vi "log analysis_gps.vi"() -> ()   [LabVIEW 2018] (continued)
INS_ALIGNMENT_COMPLETE,INS_RTKFIXED,37.37088132753,126.72154143045,8.4401,22.3000,-0.3278,-0.2536,0.0246,-0.732605001,0.589727641,213.014456450,0.4341,0.3007,0.5858,0.1132,0.0942,0.0801,0.0958,0.0999,5.1140,0f000001,0*274257ec\n\tsystem status\tnormal 2 27.800000 0 0\trobot status\t62.565143\t83.363741\t8.440100\t-0.732605\t0.589728\t-123.014456\t0.484000\t-0.004000\n\t\n15:50:00.3\tlog_raw\tgps_raw\t#INSPVAXA,USB3,0,42.0,FINESTEERING,2107,283818.350,02000000,471d,15824;INS_ALIGNMENT_COMPLETE,INS_RTKFIXED,37.37087991199,126.72154012021,8.4416,22.3000,-0.1368,-0.1470,0.0384,-0.668714112,0.493381563,212.999632348,0.4348,0.3009,0.5860,0.1136,0.0943,0.0809,0.0957,0.0999,5.1129,0f000001,0*1003161e\n\tsystem status\tnormal 2 27.800000 0 0\trobot status\t62.449084\t83.206639\t8.441600\t-0.668714\t0.493382\t-122.999632\t0.347000\t0.082000\n\t\n15:50:00.8\tlog_raw\tgps_raw\t#INSPVAXA,USB3,0,42.0,FINESTEERING,2107,283818.850,02000000,471d,15824;INS_ALIGNMENT_COMPLETE,INS_RTKFIXED,37.37087810564,126.72153855101,8.4445,22.3000,-0.4167,-0.3108,0.0271,-0.967030857,0.764287443,212.987620648,0.4348,0.3009,0.5860,0.1136,0.0943,0.0809,0.0957,0.0999,5.1129,0f000001,0*cade7f0f\n\tsystem status\tnormal 2 27.800000 0 0\trobot status\t62.310087\t83.006163\t8.444500\t-0.967031\t0.764287\t-122.987621\t0.541000\t-0.038000\n\t\n15:50:01.3\tlog_raw\tgps_raw\t\tsystem status\tnormal 2 27.700000 0 0\trobot status\t62.183899\t82.831063\t8.448200\t-1.040887\t0.633536\t-122.852792\t0.541000\t-0.102000\n\t\n15:50:01.8\tlog_raw\tgps_raw\t#INSPVAXA,USB3,0,48.0,FINESTEERING,2107,283819.850,02008000,471d,15824;INS_ALIGNMENT_COMPLETE,INS_RTKFIXED,37.37087469725,126.72153545428,8.4519,22.3000,-0.3206,-0.2482,0.0337,-0.732742938,0.483764401,213.124733025,0.4356,0.3015,0.5865,0.1140,0.0945,0.0816,0.0957,0.0999,5.1129,0f000001,0*fd809d66\n\tsystem status\tnormal 2 27.800000 0 0\trobot status\t62.035784\t82.627886\t8.451900\t-0.732743\t0.483764\t-123.124733\t0.474000\t-0.007000\n\t\n15:50:02.3\tlog_raw\tgps_raw\t#INSPVAXA,USB3,0,50.0,FINESTEERING,2107,283820.350,02008000,471d,15824;INS_ALIGNMENT_COMPLETE,INS_RTKFIXED,37.37087296887,126.72153391310,8.4559,22.3000,-0.3682,-0.2755,0.0355,-0.960553377,0.385725607,213.158574943,0.4360,0.3020,0.5871,0.1135,0.0940,0.0814,0.0957,0.0998,5.1132,0f000001,0*75b28094\n\tsystem status\tnormal 2 27.800000 0 0\trobot status\t61.899269\t82.436064\t8.455900\t-0.960553\t0.385726\t-123.158575\t0.505000\t0.011000\n\t\n15:50:02.8\tlog_raw\tgps_raw\t#INSPVAXA,USB3,0,50.0,FINESTEERING,2107,283820.850,02008000,471d,15824;INS_ALIGNMENT_COMPLETE,INS_RTKFIXED,37.37087124768,126.72153233501,8.4599,22.3000,-0.3422,-0.2623,0.0223,-0.701545718,0.294421215,213.284375134,0.4360,0.3020,0.5871,0.1135,0.0940,0.0814,0.0957,0.0998,5.1132,0f000001,0*60222fab\n\tsystem status\tnormal 2 27.800000 0 0\trobot status\t61.759484\t82.245039\t8.459900\t-0.701546\t0.294421\t-123.284375\t0.485000\t-0.013000\n\t\n15:50:03.3\tlog_raw\tgps_raw\t\tsystem status\tnormal 2 27.800000 0 0\trobot status\t61.620063\t82.053533\t8.464300\t-0.588483\t0.601593\t-123.330057\t0.501000\t-0.003000\n\t\n15:50:03.8\tlog_raw\tgps_raw\t\tsystem status\tnormal 2 27.800000 0 0\trobot status\t61.480841\t81.860839\t8.467500\t-0.490654\t0.559524\t-123.370986\t0.492000\t0.000000\n\t\n15:50:04.3\tlog_raw\tgps_raw\t#INSPVAXA,USB3,0,47.5,FINESTEERING,2107,283822.350,02008000,471d,15824;INS_ALIGNMENT_COMPLETE,INS_RTKFIXED,37.37086605631,126.72152760376,8.4704,22.3000,-0.3621,-0.2743,0.0261,-0.283958225,0.746560845,213.501890375,0.4357,0.3020,0.5877,0.1128,0.0932,0.0807,0.0958,0.0999,5.1149,0f000001,0*0669f83a\n\tsystem status\tnormal 2 27.800000 0 0\trobot status\t61.340398\t81.668880\t8.470400\t-0.283958\t0.746561\t-123.501890\t0.502000\t0.003000\n\t\n15:50:04.8\tlog_raw\tgps_raw\t#INSPVAXA,USB3,0,47.5,FINESTEERING,2107,283822.850,02008000,471d,15824;INS_ALIGNMENT_COMPLETE,INS_RTKFIXED,37.37086430536,126.72152600341,8.4729,22.3000,-0.3685,-0.2624,0.0208,-0.369026169,0.243772602,213.702415244,0.4357,0.3020,0.5877,0.1128,0.0932,0.0807,0.0958,0.0999,5.1149,0f000001,0*05a2b3f5\n\tsystem status\tnormal 2 27.800000 0 0\trobot status\t61.198641\t81.474552\t8.472900\t-0.369026\t0.243773\t-123.702415\t0.487000\t-0.013000\n\t\n15:50:05.3\tlog_raw\tgps_raw\t#INSPVAXA,USB3,0,51.5,FINESTEERING,2107,283823.350,02000000,471d,15824;INS_ALIGNMENT_COMPLETE,INS_RTKFIXED,37.37086260441,126.72152443604,8.4782,22.3000,-0.3582,-0.2656,0.0432,-0.497136063,0.605287722,213.732183523,0.4353,0.3025,0.5877,0.1126,0.0930,0.0805,0.0959,0.0999,5.1164,0f000001,0*99f3cfc8\n\tsystem status\tnormal 2 27.800000 0 0\trobot status\t61.059806\t81.285774\t8.478200\t-0.497136\t0.605288\t-123.732184\t0.485000\t-0.006000\n\t\n15:50:05.8\tlog_raw\tgps_raw\t\tsystem status\tnormal 2 27.800000 0 0\trobot status\t60.916983\t81.093453\t8.482200\t-0.454568\t0.858400\t-123.956914\t0.505000\t-0.014000\n\t\n15:50:06.3\tlog_raw\tgps_raw\t\tsystem status\tnormal 2 27.800000 0 0\trobot status\t60.774020\t80.901518\t8.486300\t-0.505119\t0.869567\t-124.073928\t0.475000\t-0.001000\n\t\n15:50:06.8\tlog_raw\tgps_raw\t\tsystem status\tnormal 2 27.800000 0 0\trobot status\t60.629827\t80.709035\t8.491500\t-0.511995\t0.882241\t-124.119289\t0.499000\t0.008000\n\t\n15:50:07.3\tlog_raw\tgps_raw\t\tsystem status\tnormal 2 27.800000 0 0\trobot status\t60.486737\t80.520026\t8.496700\t-0.379564\t1.020699\t-124.239157\t0.501000\t0.000000\n\t\n15:50:07.8\tlog_raw\tgps_raw\t\tsystem status\tnormal 2 27.800000 0 0\trobot status\t60.338417\t80.322446\t8.499300\t-0.432771\t0.777061\t-124.291372\t0.483000\t0.003000\n\t\n15:50:08.3\tlog_raw\tgps_raw\t#INSPVAXA,USB3,0,50.0,FINESTEERING,2107,283826.350,02000000,471d,15824;INS_ALIGNMENT_COMPLETE,INS_RTKFIXED,37.37085224696,126.72151466397,8.5036,22.3000,-0.3609,-0.2791,0.0409,-0.133797163,0.866362629,214.216095146,0.4345,0.3034,0.5878,0.1129,0.0936,0.0804,0.0960,0.1000,5.1194,0f000001,0*7d577a89\n\tsystem status\tnormal 2 27.700000 0 0\trobot status\t60.194212\t80.136263\t8.503600\t-0.133797\t0.866363\t-124.216095\t0.510000\t0.000000\n\t\n15:50:08.8\tlog_raw\tgps_raw\t#INSPVAXA,USB3,0,50.0,FINESTEERING,2107,283826.850,02000000,471d,15824;INS_ALIGNMENT_COMPLETE,INS_RTKFIXED,37.37085047497,126.72151297785,8.5076,22.3000,-0.3736,-0.2676,0.0140,-0.059092232,0.621746076,214.361721087,0.4345,0.3034,0.5878,0.1129,0.0936,0.0804,0.0960,0.1000,5.1194,0f000001,0*1a2aa4a2\n\tsystem status\tnormal 2 27.800000 0 0\trobot status\t60.044859\t79.939600\t8.507600\t-0.059092\t0.621746\t-124.361721\t0.500000\t0.002000\n\t\n15:50:09.3\tlog_raw\tgps_raw\t\tsystem status\tnormal 2 27.800000 0 0\trobot status\t59.900989\t79.749781\t8.510000\t-0.117922\t0.897612\t-124.301125\t0.496000\t0.007000\n\t\n15:50:09.8\tlog_raw\tgps_raw\t\tsystem status\tnormal 2 27.800000 0 0\trobot status\t59.753594\t79.555314\t8.514600\t-0.246147\t0.942410\t-124.362581\t0.504000\t0.012000\n\t\n15:50:10.3\tlog_raw\tgps_raw\t\tsystem status\tnormal 2 27.700000 0 0\trobot status\t59.607367\t79.367106\t8.518000\t-0.100537\t0.892414\t-124.256179\t0.571000\t-0.106000\n\t\n15:50:10.8\tlog_raw\tgps_raw\t#INSPVAXA,USB3,0,47.0,FINESTEERING,2107,283828.850,02000000,471d,15824;INS_ALIGNMENT_COMPLETE,INS_RTKFIXED,37.37084355919,126.72150637181,8.5210,22.3000,-0.3615,-0.2654,0.0256,-0.407156053,0.613221489,214.165441320,0.4336,0.3030,0.5876,0.1126,0.0934,0.0800,0.0960,0.1000,5.1212,0f000001,0*2be625c6\n\tsystem status\tnormal 2 27.700000 0 0\trobot status\t59.459706\t79.172059\t8.521000\t-0.407156\t0.613221\t-124.165441\t0.420000\t0.099000\n\t\n15:50:11.3\tlog_raw\tgps_raw\t\tsystem status\tnormal 2 27.800000 0 0\trobot status\t59.313902\t78.981500\t8.523300\t-0.458738\t0.721026\t-124.084724\t0.444000\t0.089000\n\t\n15:50:11.8\tlog_raw\tgps_raw\t\tsystem status\tnormal 2 27.700000 0 0\trobot status\t59.170415\t78.788865\t8.523100\t-0.646434\t0.705143\t-123.927806\t0.431000\t0.105000\n\t\n15:50:12.3\tlog_raw\tgps_raw\t\tsystem status\tnormal 2 27.800000 0 0\trobot status\t59.029369\t78.598762\t8.525600\t-0.727661\t0.618524\t-123.799711\t0.573000\t-0.111000\n\t\n15:50:12.8\tlog_raw\tgps_raw\t\tsystem status\tnormal 2 27.800000 0 0\trobot status\t58.884800\t78.404387\t8.527700\t-0.829758\t0.768744\t-123.767439\t0.440000\t0.084000\n\t\n15:50:13.3\tlog_raw\tgps_raw\t\tsystem status\tnormal 2 27.800000 0 0\trobot status\t58.743546\t78.215101\t8.526800\t-0.859789\t0.544559\t-123.753093\t0.569000\t-0.115000\n\t\n15:50:13.8\tlog_raw\tgps_raw\t\tsystem status\tnormal 2 27.800000 0 0\trobot status\t58.600898\t78.024369\t8.526600\t-0.696753\t0.469479\t-123.492403\t0.470000\t0.049000\n\t\n15:50:14.3\tlog_raw\tgps_raw\t\tsystem status\tnormal 2 27.700000 0 0\trobot status\t58.467877\t77.847457\t8.526300\t-0.753284\t0.477673\t-123.294500\t0.540000\t-0.104000\n\t\n15:50:14.8\tlog_raw\tgps_raw\t\tsystem status\tnormal 2 27.800000 0 0\trobot status\t58.320241\t77.650801\t8.527400\t-0.419843\t0.351195\t-123.324600\t0.447000\t0.018000\n\t\n15:50:15.3\tlog_raw\tgps_raw\t#INSPVAXA,USB3,0,49.5,FINESTEERING,2107,283833.350,02000000,471d,15824;INS_ALIGNMENT_COMPLETE,INS_RTKFIXED,37.37082814557,126.72149191799,8.5253,22.3000,-0.3988,-0.2653,0.0143,-0.599400887,0.523128391,213.276992929,0.4351,0.3016,0.5901,0.1136,0.0943,0.0827,0.0961,0.1001,5.1237,0f000001,0*dafc27db\n\tsystem status\tnormal 2 27.800000 0 0\trobot status\t58.179411\t77.461394\t8.525300\t-0.599401\t0.523128\t-123.276993\t0.615000\t-0.169000\n\t\n15:50:15.8\tlog_raw\tgps_raw\t\tsystem status\tnormal 2 27.700000 0 0\trobot status\t58.040086\t77.274601\t8.523600\t-0.642218\t0.408269\t-123.044870\t0.478000\t0.045000\n\t\n15:50:16.3\tlog_raw\tgps_raw\t\tsystem status\tnormal 2 27.700000 0 0\trobot status\t57.897701\t77.084219\t8.524200\t-0.645532\t0.325284\t-123.014654\t0.427000\t0.080000\n\t\n15:50:16.9\tlog_raw\tgps_raw\t\tsystem status\tnormal 2 27.800000 0 0\trobot status\t57.755522\t76.892077\t8.525700\t-0.812673\t0.258621\t-122.912534\t0.599000\t-0.151000\n\t\n15:50:17.4\tlog_raw\tgps_raw\t\tsystem status\tnormal 2 27.800000 0 0\trobot status\t57.615508\t76.704244\t8.527300\t-0.871477\t0.465364\t-122.750872\t0.437000\t0.097000\n\t\n15:50:17.8\tlog_raw\tgps_raw\t\tsystem status\tnormal 2 27.800000 0 0\trobot status\t57.474420\t76.516325\t8.527900\t-0.830453\t0.488115\t-122.693748\t0.441000\t0.077000\n\t\n15:50:18.3\tlog_raw\tgps_raw\t\tsystem status\tnormal 2 27.700000 0 0\trobot status\t57.335246\t76.328739\t8.530900\t-1.116689\t0.751675\t-122.684563\t0.468000\t0.035000\n\t\n15:50:18.9\tlog_raw\tgps_raw\t\tsystem status\tnormal 2 27.700000 0 0\trobot status\t57.194986\t76.142393\t8.532800\t-1.080685\t0.717974\t-122.524301\t0.445000\t0.006000\n\t\n15:50:19.4\tlog_raw\tgps_raw\t\tsystem status\tnormal 2 27.700000 0 0\trobot status\t57.069798\t75.976583\t8.534400\t-1.000976\t0.803716\t-122.391423\t0.541000\t0.029000\n\t\n15:50:19.9\tlog_raw\tgps_raw\t\tsystem status\tnormal 2 27.800000 0 0\trobot status\t56.929080\t75.785380\t8.534800\t-1.060163\t0.551148\t-122.452254\t0.510000\t-0.067000\n\t\n15:50:20.4\tlog_raw\tgps_raw\t\tsystem status\tnormal 2 27.800000 0 0\trobot status\t56.786562\t75.588482\t8.537500\t-1.255740\t0.371969\t-122.455535\t0.455000\t0.052000\n\t\n15:50:20.9\tlog_raw\tgps_raw\t\tsystem status\tnormal 2 27.800000 0 0\trobot status\t56.646511\t75.399961\t8.540500\t-0.936257\t0.326700\t-122.440428\t0.521000\t-0.009000\n\t\n15:50:21.4\tlog_raw\tgps_raw\t\tsystem status\tnormal 2 27.800000 0 0\trobot status\t56.509252\t75.212453\t8.543000\t-0.983282\t0.423992\t-122.415900\t0.506000\t0.009000\n\t\n15:50:21.9\tlog_raw\tgps_raw\t\tsystem status\tnormal 2 27.800000 0 0\trobot status\t56.370098\t75.020504\t8.546300\t-1.075445\t0.704997\t-122.497458\t0.489000\t0.003000\n\t\n15:50:22.4\tlog_raw\tgps_raw\t\tsystem status\tnormal 2 27.800000 0 0\trobot status\t56.230758\t74.831082\t8.551300\t-0.784818\t1.051226\t-122.242457\t0.562000\t-0.121000\n\t\n15:50:22.9\tlog_raw\tgps_raw\t\tsystem status\tnormal 2 27.700000 0 0\trobot status\t56.089782\t74.634051\t8.555400\t-0.965192\t0.771989\t-122.204085\t0.418000\t0.096000\n\t\n15:50:23.4\tlog_raw\tgps_raw\t\tsystem status\tnormal 2 27.700000 0 0\trobot status\t55.952267\t74.442660\t8.561500\t-1.095253\t0.958840\t-121.984787\t0.476000\t0.048000\n\t\n15:50:23.9\tlog_raw\tgps_raw\t\tsystem status\tnormal 2 27.800000 0 0\trobot status\t55.810060\t74.249698\t8.568200\t-0.625932\t0.756695\t-121.962841\t0.491000\t0.012000\n\t\n15:50:24.4\tlog_raw\tgps_raw\t\tsystem status\tnormal 2 27.700000 0 0\trobot status\t55.672258\t74.056371\t8.572700\t-0.978139\t0.659965\t-121.899886\t0.414000\t0.093000\n\t\n15:50:24.9\tlog_raw\tgps_raw\t\tsystem status\tnormal 2 27.800000 0 0\trobot status\t55.531120\t73.861309\t8.578200\t-0.929865\t0.602313\t-121.836312\t0.576000\t-0.107000\n\t\n15:50:25.4\tlog_raw\tgps_raw\t\tsystem status\tnormal 2 27.800000 0 0\trobot status\t55.387324\t73.664243\t8.582300\t-0.402762\t0.316758\t-121.817690\t0.484000\t0.008000\n\t\n15:50:25.9\tlog_raw\tgps_raw\t\tsystem status\tnormal 2 27.800000 0 0\trobot status\t55.250271\t73.472188\t8.586400\t-0.565675\t0.466930\t-121.851880\t0.493000\t0.003000\n\t\n15:50:26.4\tlog_raw\tgps_raw\t\tsystem status\tnormal 2 27.800000 0 0\trobot status\t55.106611\t73.274986\t8.590300\t-0.388856\t0.450311\t-121.847107\t0.444000\t0.085000\n\t\n15:50:26.9\tlog_raw\tgps_raw\t\tsystem status\tnormal 2 27.700000 0 0\trobot status\t54.967816\t73.083854\t8.595900\t-0.079145\t0.424625\t-121.735110\t0.471000\t0.030000\n\t\n15:50:27.4\tlog_raw\tgps_raw\t\tsystem status\tnormal 2 27.800000 0 0\trobot status\t54.826021\t72.881844\t8.600700\t-0.151083\t0.220851\t-121.840766\t0.513000\t-0.009000\n\t\n15:50:27.9\tlog_raw\tgps_raw\t\tsystem status\tnormal 2 27.800000 0 0\trobot status\t54.690256\t72.690886\t8.605600\t-0.106460\t0.706261\t-121.827652\t0.496000\t-0.004000\n\t\n15:50:28.4\tlog_raw\tgps_raw\t\tsystem status\tnormal 2 27.800000 0 0\trobot status\t54.549384\t72.491140\t8.608600\t-0.035331\t0.689454\t-121.793907\t0.497000\t-0.005000\n\t\n15:50:28.9\tlog_raw\tgps_raw\t\tsystem status\tnormal 2 27.800000 0 0\trobot status\t54.413442\t72.300322\t8.613400\t-0.074908\t0.770755\t-121.742164\t0.492000\t0.012000\n\t\n15:50:29.4\tlog_raw\tgps_raw\t\tsystem status\tnormal 2 27.800000 0 0\trobot status\t54.275777\t72.104249\t8.621100\t-0.231468\t0.799148\t-121.909740\t0.506000\t-0.009000\n\t\n15:50:29.9\tlog_raw\tgps_raw\t#INSPVAXA,USB3,0,51.5,FINESTEERING,2107,283847.900,02000000,471d,15824;INS_ALIGNMENT_COMPLETE,INS_RTKFIXED,37.37077798648,126.72144617612,8.6277,22.3000,-0.3813,-0.2770,0.0286,-0.218735739,0.822253725,211.859941742,0.4334,0.3030,0.5894,0.1137,0.0946,0.0820,0.0959,0.1000,5.1292,0f000001,0*a6b72ce6\n\tsystem status\tnormal 2 27.800000 0 0\trobot status\t54.127671\t71.894534\t8.627700\t-0.218736\t0.822254\t-121.859942\t0.547000\t-0.101000\n\t\n15:50:30.4\tlog_raw\tgps_raw\t\tsystem status\tnormal 2 27.800000 0 0\trobot status\t54.003309\t71.718655\t8.634300\t-0.094224\t0.760414\t-121.875157\t0.492000\t-0.011000\n\t\n15:50:30.9\tlog_raw\tgps_raw\t\tsystem status\tnormal 2 27.800000 0 0\trobot status\t53.865381\t71.521678\t8.640700\t-0.318590\t0.754266\t-121.881064\t0.538000\t-0.051000\n\t\n15:50:31.4\tlog_raw\tgps_raw\t#INSPVAXA,USB3,0,50.5,FINESTEERING,2107,283849.400,02000000,471d,15824;INS_ALIGNMENT_COMPLETE,INS_RTKFIXED,37.37077272118,126.72144151665,8.6465,22.3000,-0.4175,-0.3003,0.0168,-0.333999296,0.525608406,211.832287674,0.4333,0.3042,0.5899,0.1136,0.0946,0.0824,0.0960,0.1001,5.1298,0f000001,0*7349f925\n\tsystem status\tnormal 2 27.800000 0 0\trobot status\t53.714943\t71.310170\t8.646500\t-0.333999\t0.525608\t-121.832288\t0.505000\t0.007000\n\t\n15:50:31.9\tlog_raw\tgps_raw\t\tsystem status\tnormal 2 27.700000 0 0\trobot status\t53.591445\t71.140770\t8.651200\t-0.196955\t0.528044\t-121.860602\t0.517000\t-0.036000\n\t\n15:50:32.4\tlog_raw\tgps_raw\t\tsystem status\tnormal 2 27.800000 0 0\trobot status\t53.453573\t70.944417\t8.655800\t-0.428339\t0.453425\t-121.948264\t0.493000\t-0.002000\n\t\n15:50:32.9\tlog_raw\tgps_raw\t#INSPVAXA,USB3,0,41.0,FINESTEERING,2107,283850.900,02000000,471d,15824;INS_ALIGNMENT_COMPLETE,INS_RTKFIXED,37.37076749535,126.72143686208,8.6606,22.3000,-0.3847,-0.2816,0.0281,-0.406598384,0.513432483,212.015462221,0.4333,0.3045,0.5903,0.1132,0.0939,0.0820,0.0961,0.1001,5.1303,0f000001,0*8e06507b\n\tsystem status\tnormal 2 27.800000 0 0\trobot status\t53.302648\t70.730186\t8.660600\t-0.406598\t0.513432\t-122.015462\t0.494000\t0.000000\n\t\n15:50:33.4\tlog_raw\tgps_raw\t\tsystem status\tnormal 2 27.800000 0 0\trobot status\t53.184999\t70.564620\t8.665200\t-0.348900\t0.522368\t-121.871475\t0.518000\t-0.029000\n\t\n15:50:33.9\tlog_raw\tgps_raw\t\tsystem status\tnormal 2 27.800000 0 0\trobot status\t53.046174\t70.369116\t8.670700\t-0.320105\t0.727759\t-122.063167\t0.485000\t0.003000\n\t\n15:50:34.4\tlog_raw\tgps_raw\t\tsystem status\tnormal 2 27.800000 0 0\trobot status\t52.912069\t70.180872\t8.675300\t-0.303842\t0.847914\t-122.052980\t0.493000\t-0.011000\n\t\n15:50:34.9\tlog_raw\tgps_raw\t\tsystem status\tnormal 2 27.800000 0 0\trobot status\t52.774733\t69.989489\t8.683800\t-0.202462\t0.682142\t-122.083895\t0.498000\t-0.013000\n\t\n15:50:35.4\tlog_raw\tgps_raw\t\tsystem status\tnormal 2 27.800000 0 0\trobot status\t52.640255\t69.801096\t8.691800\t-0.326948\t1.068096\t-122.130007\t0.487000\t0.004000\n\t\n15:50:35.9\tlog_raw\tgps_raw\t\tsystem status\tnormal 2 27.800000 0 0\trobot status\t52.504199\t69.611397\t8.698900\t-0.226041\t0.917411\t-122.099016\t0.488000\t0.005000\n\t\n15:50:36.4\tlog_raw\tgps_raw\t#INSPVAXA,USB3,0,51.0,FINESTEERING,2107,283854.400,02000000,471d,15824;INS_ALIGNMENT_COMPLETE,INS_RTKFIXED,37.37075554514,126.72142617070,8.7046,22.3000,-0.3702,-0.2734,0.0406,-0.208946462,1.069935168,212.200844813,0.4356,0.3041,0.5961,0.1134,0.0944,0.0821,0.0963,0.1002,5.1349,0f000001,0*eaf32da8\n\tsystem status\tnormal 2 27.800000 0 0\trobot status\t52.355623\t69.403902\t8.704600\t-0.208946\t1.069935\t-122.200845\t0.495000\t-0.006000\n\t\n15:50:36.9\tlog_raw\tgps_raw\t\tsystem status\tnormal 2 27.800000 0 0\trobot status\t52.233569\t69.230205\t8.708800\t-0.301434\t0.977951\t-122.256655\t0.514000\t-0.006000\n\t\n15:50:37.4\tlog_raw\tgps_raw\t#INSPVAXA,USB3,0,52.5,FINESTEERING,2107,283855.400,02000000,471d,15824;INS_ALIGNMENT_COMPLETE,INS_RTKFIXED,37.37075208909,126.72142312545,8.7152,22.3000,-0.3888,-0.2785,0.0279,-0.502124880,0.807271282,212.351278454,0.4348,0.3040,0.5953,0.1133,0.0940,0.0816,0.0963,0.1002,5.1361,0f000001,0*26b77d4e\n\tsystem status\tnormal 2 27.800000 0 0\trobot status\t52.085880\t69.020336\t8.715200\t-0.502125\t0.807271\t-122.351278\t0.487000\t-0.009000\n\t\n15:50:37.9\tlog_raw\tgps_raw\t#INSPVAXA,USB3,0,52.5,FINESTEERING,2107,283855.900,02000000,471d,15824;INS_ALIGNMENT_COMPLETE,INS_RTKFIXED,37.37075038942,126.72142158334,8.7226,22.3000,-0.3755,-0.2603,0.0501,-0.282397240,0.801872583,212.409267402,0.4348,0.3040,0.5953,0.1133,0.0940,0.0816,0.0963,0.1002,5.1361,0f000001,0*7c1b1b61\n\tsystem status\tnormal 2 27.800000 0 0\trobot status\t51.949283\t68.831699\t8.722600\t-0.282397\t0.801873\t-122.409267\t0.499000\t0.005000\n\t\n15:50:38.4\tlog_raw\tgps_raw\t#INSPVAXA,USB3,0,53.5,FINESTEERING,2107,283856.400,02000000,471d,15824;INS_ALIGNMENT_COMPLETE,INS_RTKFIXED,37.37074865373,126.72142004246,8.7267,22.3000,-0.3704,-0.2786,0.0171,-0.353111883,0.600799682,212.485026381,0.4344,0.3035,0.5945,0.1128,0.0938,0.0812,0.0963,0.1002,5.1372,0f000001,0*81e7853e\n\tsystem status\tnormal 2 27.800000 0 0\trobot status\t51.812794\t68.639065\t8.726700\t-0.353112\t0.600800\t-122.485026\t0.488000\t-0.004000\n\t\n15:50:38.9\tlog_raw\tgps_raw\t#INSPVAXA,USB3,0,53.5,FINESTEERING,2107,283856.900,02000000,471d,15824;INS_ALIGNMENT_COMPLETE,INS_RTKFIXED,37.37074693319,126.72141850353,8.7310,22.3000,-0.3735,-0.2746,0.0382,-0.533241802,0.632806035,212.664304846,0.4344,0.3035,0.5945,0.1128,0.0938,0.0812,0.0963,0.1002,5.1372,0f000001,0*a05af5ad\n\tsystem status\tnormal 2 27.800000 0 0\trobot status\t51.676478\t68.448113\t8.731000\t-0.533242\t0.632806\t-122.664305\t0.486000\t-0.012000\n\t\n15:50:39.4\tlog_raw\tgps_raw\t#INSPVAXA,USB3,0,49.5,FINESTEERING,2107,283857.400,02000000,471d,15824;INS_ALIGNMENT_COMPLETE,INS_RTKFIXED,37.37074522542,126.72141694545,8.7353,22.3000,-0.3672,-0.2584,0.0083,-0.503263302,0.873939693,212.796225094,0.4338,0.3028,0.5936,0.1126,0.0936,0.0808,0.0963,0.1002,5.1384,0f000001,0*83ef516a\n\tsystem status\tnormal 2 27.800000 0 0\trobot status\t51.538466\t68.258577\t8.735300\t-0.503263\t0.873940\t-122.796225\t0.490000\t-0.009000\n\t\n15:50:39.9\tlog_raw\tgps_raw\t\tsystem status\tnormal 2 27.800000 0 0\trobot status\t51.414123\t68.086719\t8.738100\t-0.575490\t0.860544\t-122.909688\t0.498000\t0.006000\n\t\n15:50:40.4\tlog_raw\tgps_raw\t#INSPVAXA,USB3,0,48.5,FINESTEERING,2107,283858.400,02000000,471d,15824;INS_ALIGNMENT_COMPLETE,INS_RTKFIXED,37.37074181137,126.72141381926,8.7415,22.3000,-0.3728,-0.3056,0.0242,-0.533104830,1.057002190,212.963002885,0.4334,0.3023,0.5928,0.1134,0.0944,0.0817,0.0962,0.1002,5.1397,0f000001,0*eea1e126\n\tsystem status\tnormal 2 27.800000 0 0\trobot status\t51.261553\t67.879672\t8.741500\t-0.533105\t1.057002\t-122.963003\t0.504000\t0.007000\n\t\n15:50:40.9\tlog_raw\tgps_raw\t#INSPVAXA,USB3,0,48.5,FINESTEERING,2107,283858.900,02000000,471d,15824;INS_ALIGNMENT_COMPLETE,INS_RTKFIXED,37.37074011417,126.72141223787,8.7461,22.3000,-0.3747,-0.2786,0.0449,-0.561180315,0.752123246,213.105436806,0.4334,0.3023,0.5928,0.1134,0.0944,0.0817,0.0962,0.1002,5.1397,0f000001,0*c4922269\n\tsystem status\tnormal 2 27.800000 0 0\trobot status\t51.121476\t67.691310\t8.746100\t-0.561180\t0.752123\t-123.105437\t0.485000\t-0.018000\n\t\n15:50:41.4\tlog_raw\tgps_raw\t\tsystem status\tnormal 2 27.800000 0 0\trobot status\t50.995151\t67.518763\t8.750800\t-0.701801\t0.945703\t-123.228772\t0.492000\t-0.004000\n\t\n15:50:41.9\tlog_raw\tgps_raw\t#INSPVAXA,USB3,0,46.0,FINESTEERING,2107,283859.900,02000000,471d,15824;INS_ALIGNMENT_COMPLETE,INS_RTKFIXED,37.37073667123,126.72140904709,8.7547,22.3000,-0.3866,-0.2889,0.0316,-0.473578727,0.831151381,213.327049680,0.4335,0.3024,0.5921,0.1137,0.0949,0.0823,0.0962,0.1002,5.1407,0f000001,0*c02ad3f9\n\tsystem status\tnormal 2 27.800000 0 0\trobot status\t50.838842\t67.309198\t8.754700\t-0.473579\t0.831151\t-123.327050\t0.495000\t-0.006000\n\t\n15:50:42.4\tlog_raw\tgps_raw\t#INSPVAXA,USB3,0,48.5,FINESTEERING,2107,283860.400,02000000,471d,15824;INS_ALIGNMENT_COMPLETE,INS_RTKFIXED,37.37073499313,126.72140747004,8.7594,22.3000,-0.3720,-0.2575,0.0488,-0.469904775,1.004834179,213.445822894,0.4337,0.3023,0.5918,0.1139,0.0949,0.0827,0.0962,0.1002,5.1415,0f000001,0*acdd0918\n\tsystem status\tnormal 2 27.800000 0 0\trobot status\t50.699150\t67.122956\t8.759400\t-0.469905\t1.004834\t-123.445823\t0.492000\t0.000000\n\t\n15:50:42.9\tlog_raw\tgps_raw\t\tsystem status\tnormal 2 27.800000 0 0\trobot status\t50.572215\t66.954306\t8.763600\t-0.540791\t1.123928\t-123.475423\t0.490000\t-0.002000\n\t\n15:50:43.4\tlog_raw\tgps_raw\t#INSPVAXA,USB3,0,51.0,FINESTEERING,2107,283861.400,02000000,471d,15824;INS_ALIGNMENT_COMPLETE,INS_RTKFIXED,37.37073158735,126.72140425235,8.7667,22.3000,-0.3807,-0.2830,0.0264,-0.516210475,0.946045536,213.526350535,0.4337,0.3025,0.5918,0.1135,0.0942,0.0822,0.0962,0.1002,5.1424,0f000001,0*0628bfaf\n\tsystem status\tnormal 2 27.800000 0 0\trobot status\t50.414132\t66.744969\t8.766700\t-0.516210\t0.946046\t-123.526351\t0.501000\t0.000000\n\t\n15:50:43.9\tlog_raw\tgps_raw\t#INSPVAXA,USB3,0,51.0,FINESTEERING,2107,283861.900,02000000,471d,15824;INS_ALIGNMENT_COMPLETE,INS_RTKFIXED,37.37072989036,126.72140267058,8.7698,22.3000,-0.3805,-0.2823,0.0328,-0.596244967,0.822145304,213.518686009,0.4337,0.3025,0.5918,0.1135,0.0942,0.0822,0.0962,0.1002,5.1424,0f000001,0*59f9b731\n\tsystem status\tnormal 2 27.800000 0 0\trobot status\t50.274021\t66.556630\t8.769800\t-0.596245\t0.822145\t-123.518686\t0.492000\t-0.001000\n\t\n15:50:44.4\tlog_raw\tgps_raw\t\tsystem status\tnormal 2 27.800000 0 0\trobot status\t50.145474\t66.384572\t8.772300\t-0.494772\t0.636142\t-123.530677\t0.497000\t0.016000\n\t\n15:50:44.9\tlog_raw\tgps_raw\t#INSPVAXA,USB3,0,53.5,FINESTEERING,2107,283862.900,02000000,471d,15824;INS_ALIGNMENT_COMPLETE,INS_RTKFIXED,37.37072646005,126.72139945545,8.7731,22.3000,-0.3733,-0.2791,0.0108,-0.480391317,0.493865630,213.689633604,0.4337,0.3029,0.5918,0.1135,0.0944,0.0825,0.0962,0.1002,5.1434,0f000001,0*a4999ec0\n\tsystem status\tnormal 2 27.800000 0 0\trobot status\t49.989230\t66.175920\t8.773100\t-0.480391\t0.493866\t-123.689634\t0.514000\t-0.009000\n\t\n15:50:45.4\tlog_raw\tgps_raw\t#INSPVAXA,USB3,0,51.0,FINESTEERING,2107,283863.400,02000000,471d,15824;INS_ALIGNMENT_COMPLETE,INS_RTKFIXED,37.37072475302,126.72139787824,8.7760,22.3000,-0.3764,-0.2596,0.0258,-0.739706001,0.670082501,213.669288600,0.4337,0.3025,0.5920,0.1136,0.0946,0.0829,0.0962,0.1002,5.1442,0f000001,0*2644d37e\n\tsystem status\tnormal 2 27.800000 0 0\trobot status\t49.849524\t65.986466\t8.776000\t-0.739706\t0.670083\t-123.669289\t0.499000\t-0.007000\n\t\n15:50:45.9\tlog_raw\tgps_raw\t#INSPVAXA,USB3,0,51.0,FINESTEERING,2107,283863.900,02000000,471d,15824;INS_ALIGNMENT_COMPLETE,INS_RTKFIXED,37.37072304752,126.72139625186,8.7774,22.3000,-0.3739,-0.2776,0.0095,-0.592048813,0.512858397,213.725097807,0.4337,0.3025,0.5920,0.1136,0.0946,0.0829,0.0962,0.1002,5.1442,0f000001,0*9580d57a\n\tsystem status\tnormal 2 27.800000 0 0\trobot status\t49.705462\t65.797183\t8.777400\t-0.592049\t0.512858\t-123.725098\t0.500000\t-0.001000\n\t\n15:50:46.4\tlog_raw\tgps_raw\t#INSPVAXA,USB3,0,48.5,FINESTEERING,2107,283864.400,02000000,471d,15824;INS_ALIGNMENT_COMPLETE,INS_RTKFIXED,37.37072134638,126.72139464126,8.7780,22.3000,-0.3662,-0.2725,0.0206,-0.511623152,0.752820747,213.729098110,0.4338,0.3024,0.5923,0.1139,0.0949,0.0834,0.0963,0.1002,5.1449,0f000001,0*0ef3aee0\n\tsystem status\tnormal 2 27.800000 0 0\trobot status\t49.562797\t65.608384\t8.778000\t-0.511623\t0.752821\t-123.729098\t0.481000\t0.007000\n\t\n15:50:46.9\tlog_raw\tgps_raw\t#INSPVAXA,USB3,0,48.5,FINESTEERING,2107,283864.900,02000000,471d,15824;INS_ALIGNMENT_COMPLETE,INS_RTKFIXED,37.37071966406,126.72139308465,8.7791,22.3000,-0.2990,-0.2177,0.0217,-0.848822059,0.608273081,213.821443632,0.4338,0.3024,0.5923,0.1139,0.0949,0.0834,0.0963,0.1002,5.1449,0f000001,0*1bce49ab\n\tsystem status\tnormal 2 27.800000 0 0\trobot status\t49.424915\t65.421673\t8.779100\t-0.848822\t0.608273\t-123.821444\t0.321000\t0.019000\n\t\n15:50:47.4\tlog_raw\tgps_raw\t#INSPVAXA,USB3,0,51.0,FINESTEERING,2107,283865.400,02000000,471d,15824;INS_ALIGNMENT_COMPLETE,INS_RTKFIXED,37.37071856255,126.72139199889,8.7824,22.3000,-0.5108,-0.3655,0.0313,-0.933274123,1.127883317,213.366579134,0.4336,0.3023,0.5928,0.1148,0.0954,0.0839,0.0963,0.1002,5.1456,0f000001,0*e5b04468\n\tsystem status\tnormal 2 27.500000 0 0\trobot status\t49.328741\t65.299423\t8.782400\t-0.933274\t1.127883\t-123.366579\t0.542000\t0.025000\n\t\n15:50:47.9\tlog_raw\tgps_raw\t#INSPVAXA,USB3,0,51.0,FINESTEERING,2107,283865.900,02000000,471d,15824;INS_ALIGNMENT_COMPLETE,INS_RTKFIXED,37.37071661051,126.72139019548,8.7866,22.3000,-0.2777,-0.2015,0.0278,-1.149054728,0.648107164,213.765006412,0.4336,0.3023,0.5928,0.1148,0.0954,0.0839,0.0963,0.1002,5.1456,0f000001,0*0fe651af\n\tsystem status\tnormal 2 27.800000 0 0\trobot status\t49.168997\t65.082777\t8.786600\t-1.149055\t0.648107\t-123.765006\t0.575000\t-0.115000\n\t\n15:50:48.4\tlog_raw\tgps_raw\t#INSPVAXA,USB3,0,51.0,FINESTEERING,2107,283866.400,02000000,471d,15824;INS_ALIGNMENT_COMPLETE,INS_RTKFIXED,37.37071495847,126.72138864071,8.7911,22.3000,-0.4383,-0.3177,0.0305,-1.188306881,0.667471315,213.730398031,0.4343,0.3039,0.5934,0.1144,0.0951,0.0843,0.0964,0.1003,5.1466,0f000001,0*5b447a13\n\tsystem status\tnormal 2 27.700000 0 0\trobot status\t49.031278\t64.899427\t8.791100\t-1.188307\t0.667471\t-123.730398\t0.539000\t-0.025000\n\t\n15:50:48.9\tlog_raw\tgps_raw\t#INSPVAXA,USB3,0,51.0,FINESTEERING,2107,283866.900,02000000,471d,15824;INS_ALIGNMENT_COMPLETE,INS_RTKFIXED,37.37071327557,126.72138707282,8.7965,22.3000,-0.3634,-0.2672,0.0089,-1.371908474,0.653216644,213.825388529,0.4343,0.3039,0.5934,0.1144,0.0951,0.0843,0.0964,0.1003,5.1466,0f000001,0*b2617258\n\tsystem status\tnormal 2 27.800000 0 0\trobot status\t48.892397\t64.712652\t8.796500\t-1.371908\t0.653217\t-123.825389\t0.474000\t0.003000\n\t\n15:50:49.4\tlog_raw\tgps_raw\t#INSPVAXA,USB3,0,52.0,FINESTEERING,2107,283867.400,02000000,471d,15824;INS_ALIGNMENT_COMPLETE,INS_RTKFIXED,37.37071150650,126.72138537987,8.7986,22.3000,-0.3586,-0.2741,0.0372,-1.171252823,0.553114037,213.926060837,0.4346,0.3035,0.5942,0.1136,0.0954,0.0837,0.0964,0.1003,5.1472,0f000001,0*449ce9b9\n\tsystem status\tnormal 2 27.800000 0 0\trobot status\t48.742439\t64.516313\t8.798600\t-1.171253\t0.553114\t-123.926061\t0.516000\t-0.005000\n\t\n15:50:49.9\tlog_raw\tgps_raw\t#INSPVAXA,USB3,0,52.0,FINESTEERING,2107,283867.900,02000000,471d,15824;INS_ALIGNMENT_COMPLETE,INS_RTKFIXED,37.37070986171,126.72138379312,8.8042,22.3000,-0.3895,-0.2987,0.0305,-0.968121893,0.950264581,213.826020130,0.4346,0.3035,0.5942,0.1136,0.0954,0.0837,0.0964,0.1003,5.1472,0f000001,0*7d4cf138\n\tsystem status\tnormal 2 27.700000 0 0\trobot status\t48.601887\t64.333768\t8.804200\t-0.968122\t0.950265\t-123.826020\t0.503000\t0.003000\n\t\n15:50:50.4\tlog_raw\tgps_raw\t#INSPVAXA,USB3,0,53.5,FINESTEERING,2107,283868.400,02000000,471d,15824;INS_ALIGNMENT_COMPLETE,INS_RTKFIXED,37.37070816169,126.72138212704,8.8085,22.3000,-0.3715,-0.2818,0.0239,-0.767361494,1.034807260,213.960421110,0.4345,0.3021,0.5949,0.1138,0.0953,0.0840,0.0965,0.1004,5.1465,0f000001,0*55731318\n\tsystem status\tnormal 2 27.800000 0 0\trobot status\t48.454308\t64.145093\t8.808500\t-0.767361\t1.034807\t-123.960421\t0.495000\t0.006000\n\t\n15:50:50.9\tlog_raw\tgps_raw\t#DUALANTENNAHEADINGA,USB3,0,53.5,FINESTEERING,2107,283868.900,02000000,d426,15824;INSUFFICIENT_OBS,NONE,-1.000000000,0.000000000,0.000000000,0.0,0.000000000,0.000000000,\"631T\",14,3,3,3,04,00,20,00*2bda417b\n\tsystem status\tnormal 2 27.800000 0 0\trobot status\t48.309383\t63.958566\t8.812500\t-0.802388\t1.025902\t-124.001232\t0.480000\t0.009000\n\t\n15:50:51.4\tlog_raw\tgps_raw\t#INSPVAXA,USB3,0,47.5,FINESTEERING,2107,283869.400,02000000,471d,15824;INS_ALIGNMENT_COMPLETE,INS_RTKFIXED,37.37070477498,126.72137878954,8.8182,22.3000,-0.3794,-0.2856,0.0387,-0.580248712,0.693765436,214.050059591,0.4343,0.3016,0.5953,0.1139,0.0951,0.0843,0.0965,0.1004,5.1447,0f000001,0*5005ba7a\n\tsystem status\tnormal 2 27.800000 0 0\trobot status\t48.158678\t63.769222\t8.818200\t-0.580249\t0.693765\t-124.050060\t0.500000\t-0.003000\n\t\n15:50:51.9\tlog_raw\tgps_raw\t#INSPVAXA,USB3,0,47.5,FINESTEERING,2107,283869.900,02000000,471d,15824;INS_ALIGNMENT_COMPLETE,INS_RTKFIXED,37.37070349907,126.72137747347,8.8234,22.3000,-0.3765,-0.2687,0.0325,-0.595922163,0.823980271,213.804726387,0.4343,0.3016,0.5953,0.1139,0.0951,0.0843,0.0965,0.1004,5.1447,0f000001,0*b08e18e5\n\tsystem status\tnormal 2 27.600000 0 0\trobot status\t48.042103\t63.627616\t8.823400\t-0.595922\t0.823980\t-123.804726\t0.440000\t-0.016000\n\t\n15:50:52.4\tlog_raw\tgps_raw\t#INSPVAXA,USB3,0,48.0,FINESTEERING,2107,283870.400,02000000,471d,15824;INS_ALIGNMENT_COMPLETE,INS_RTKFIXED,37.37070163427,126.72137570159,8.8300,22.3000,-0.3041,-0.2407,0.0180,-0.604642888,0.778196285,214.030795943,0.4340,0.3016,0.5956,0.1141,0.0959,0.0845,0.0966,0.1004,5.1433,0f000001,0*cb822ea1\n\tsystem status\tnormal 2 27.800000 0 0\trobot status\t47.885152\t63.420653\t8.830000\t-0.604643\t0.778196\t-124.030796\t0.455000\t0.058000\n\t\n15:50:52.9\tlog_raw\tgps_raw\t#INSPVAXA,USB3,0,48.0,FINESTEERING,2107,283870.900,02000000,471d,15824;INS_ALIGNMENT_COMPLETE,INS_RTKFIXED,37.37069994386,126.72137408130,8.8327,22.3000,-0.4129,-0.3185,0.0299,-0.561714396,1.101086671,213.985768500,0.4340,0.3016,0.5956,0.1141,0.0959,0.0845,0.0966,0.1004,5.1433,0f000001,0*097c1e24\n\tsystem status\tnormal 2 27.800000 0 0\trobot status\t47.741630\t63.233044\t8.832700\t-0.561714\t1.101087\t-123.985769\t0.533000\t-0.006000\n\t\n15:50:53.4\tlog_raw\tgps_raw\t#INSPVAXA,USB3,0,50.0,FINESTEERING,2107,283871.400,02000000,471d,15824;INS_ALIGNMENT_COMPLETE,INS_RTKFIXED,37.37069831939,126.72137250494,8.8386,22.3000,-0.3879,-0.3050,0.0340,-0.603840717,0.986135442,213.822522610,0.4341,0.3014,0.5961,0.1146,0.0956,0.0852,0.0966,0.1005,5.1404,0f000001,0*99650335\n\tsystem status\tnormal 2 27.800000 0 0\trobot status\t47.601998\t63.052754\t8.838600\t-0.603841\t0.986135\t-123.822523\t0.493000\t0.021000\n\t\n15:50:53.9\tlog_raw\tgps_raw\t#INSPVAXA,USB3,0,50.0,FINESTEERING,2107,283871.900,02000000,471d,15824;INS_ALIGNMENT_COMPLETE,INS_RTKFIXED,37.37069663076,126.72137084332,8.8454,22.3000,-0.3570,-0.2814,0.0330,-0.426296070,0.946461964,213.763011209,0.4341,0.3014,0.5961,0.1146,0.0956,0.0852,0.0966,0.1005,5.1404,0f000001,0*8cc6f2c5\n\tsystem status\tnormal 2 27.700000 0 0\trobot status\t47.454815\t62.865343\t8.845400\t-0.426296\t0.946462\t-123.763011\t0.467000\t0.028000\n\t\n15:50:54.4\tlog_raw\tgps_raw\t#INSPVAXA,USB3,0,48.5,FINESTEERING,2107,283872.400,02000000,471d,15824;INS_ALIGNMENT_COMPLETE,INS_RTKFIXED,37.37069491831,126.72136922755,8.8525,22.3000,-0.3761,-0.2771,0.0323,-0.638578544,0.908546721,213.728365329,0.4343,0.3024,0.5968,0.1148,0.0958,0.0857,0.0966,0.1006,5.1403,0f000001,0*b6cc0c4e\n\tsystem status\tnormal 2 27.700000 0 0\trobot status\t47.311693\t62.675288\t8.852500\t-0.638579\t0.908547\t-123.728365\t0.455000\t0.049000\n\t\n15:50:54.9\tlog_raw\tgps_raw\t#INSPVAXA,USB3,0,48.5,FINESTEERING,2107,283872.900,02000000,471d,15824;INS_ALIGNMENT_COMPLETE,INS_RTKFIXED,37.37069321684,126.72136760945,8.8593,22.3000,-0.3790,-0.2963,0.0419,-0.436104629,0.871418994,213.562317886,0.4343,0.3024,0.5968,0.1148,0.0958,0.0857,0.0966,0.1006,5.1403,0f000001,0*c4a88a6a\n\tsystem status\tnormal 2 27.700000 0 0\trobot status\t47.168364\t62.486452\t8.859300\t-0.436105\t0.871419\t-123.562318\t0.620000\t-0.156000\n\t\n15:50:55.4\tlog_raw\tgps_raw\t#INSPVAXA,USB3,0,49.5,FINESTEERING,2107,283873.400,02008000,471d,15824;INS_ALIGNMENT_COMPLETE,INS_RTKFIXED,37.37069152716,126.72136602353,8.8633,22.3000,-0.3871,-0.2959,0.0071,-0.372350545,0.744743761,213.502289859,0.4348,0.3034,0.5975,0.1151,0.0961,0.0863,0.0967,0.1006,5.1413,0f000001,0*db4d8b18\n\tsystem status\tnormal 2 27.700000 0 0\trobot status\t47.027886\t62.298924\t8.863300\t-0.372351\t0.744744\t-123.502290\t0.577000\t-0.102000\n\t\n15:50:55.9\tlog_raw\tgps_raw\t#INSPVAXA,USB3,0,49.5,FINESTEERING,2107,283873.900,02008000,471d,15824;INS_ALIGNMENT_COMPLETE,INS_RTKFIXED,37.37068980188,126.72136442451,8.8669,22.3000,-0.3821,-0.2876,0.0223,-0.542252908,0.493927279,213.372683943,0.4348,0.3034,0.5975,0.1151,0.0961,0.0863,0.0967,0.1006,5.1413,0f000001,0*34acffbe\n\tsystem status\tnormal 2 27.800000 0 0\trobot status\t46.886247\t62.107445\t8.866900\t-0.542253\t0.493927\t-123.372684\t0.473000\t0.018000\n\t\n15:50:56.4\tlog_raw\tgps_raw\t#INSPVAXA,USB3,0,52.5,FINESTEERING,2107,283874.400,02008000,471d,15824;INS_ALIGNMENT_COMPLETE,INS_RTKFIXED,37.37068808694,126.72136282059,8.8713,22.3000,-0.3710,-0.2644,0.0357,-0.579423021,0.489216985,213.355766858,0.4351,0.3041,0.5984,0.1155,0.0964,0.0870,0.0968,0.1007,5.1427,0f000001,0*1b568777\n\tsystem status\tnormal 2 27.800000 0 0\trobot status\t46.744175\t61.917114\t8.871300\t-0.579423\t0.489217\t-123.355767\t0.463000\t0.059000\n\t\n15:50:56.9\tlog_raw\tgps_raw\t#DUALANTENNAHEADINGA,USB3,0,52.5,FINESTEERING,2107,283874.900,02008000,d426,15824;INSUFFICIENT_OBS,NONE,-1.000000000,0.000000000,0.000000000,0.0,0.000000000,0.000000000,\"631T\",11,3,3,3,04,00,20,00*2cd613df\n\tsystem status\tnormal 2 27.800000 0 0\trobot status\t46.601872\t61.730059\t8.878300\t-0.397886\t0.409795\t-123.234520\t0.483000\t0.032000\n\t\n15:50:57.4\tlog_raw\tgps_raw\t#INSPVAXA,USB3,0,49.5,FINESTEERING,2107,283875.400,02008000,471d,15824;INS_ALIGNMENT_COMPLETE,INS_RTKFIXED,37.37068468930,126.72135963115,8.8825,22.3000,-0.3622,-0.2842,0.0299,-0.576500581,0.429092334,213.280984070,0.4354,0.3044,0.5994,0.1156,0.0965,0.0875,0.0969,0.1007,5.1441,0f000001,0*e8de9d75\n\tsystem status\tnormal 2 27.700000 0 0\trobot status\t46.461659\t61.540030\t8.882500\t-0.576501\t0.429092\t-123.280984\t0.436000\t0.071000\n\t\n15:50:57.9\tlog_raw\tgps_raw\t#INSPVAXA,USB3,0,49.5,FINESTEERING,2107,283875.900,02008000,471d,15824;INS_ALIGNMENT_COMPLETE,INS_RTKFIXED,37.37068297802,126.72135803904,8.8854,22.3000,-0.3707,-0.2810,0.0365,-0.547997166,0.698496112,213.263606551,0.4354,0.3044,0.5994,0.1156,0.0965,0.0875,0.0969,0.1007,5.1441,0f000001,0*65e2a656\n\tsystem status\tnormal 2 27.800000 0 0\trobot status\t46.320633\t61.350105\t8.885400\t-0.547997\t0.698496\t-123.263607\t0.507000\t0.004000\n\t\n15:50:58.4\tlog_raw\tgps_raw\t#INSPVAXA,USB3,0,44.0,FINESTEERING,2107,283876.400,02008000,471d,15824;INS_ALIGNMENT_COMPLETE,INS_RTKFIXED,37.37068125444,126.72135642974,8.8888,22.3000,-0.3786,-0.2878,0.0233,-0.531966030,0.387673420,213.289464944,0.4359,0.3047,0.6005,0.1161,0.0970,0.0885,0.0969,0.1008,5.1456,0f000001,0*b4409e90\n\tsystem status\tnormal 2 27.800000 0 0\trobot status\t46.178084\t61.158815\t8.888800\t-0.531966\t0.387673\t-123.289465\t0.494000\t0.000000\n\t\n15:50:58.9\tlog_raw\tgps_raw\t#INSPVAXA,USB3,0,44.0,FINESTEERING,2107,283876.900,02008000,471d,15824;INS_ALIGNMENT_COMPLETE,INS_RTKFIXED,37.37067957761,126.72135484740,8.8937,22.3000,-0.4026,-0.3012,0.0273,-0.420783044,0.494040879,213.316912941,0.4359,0.3047,0.6005,0.1161,0.0970,0.0885,0.0969,0.1008,5.1456,0f000001,0*00e3c1db\n\tsystem status\tnormal 2 27.800000 0 0\trobot status\t46.037922\t60.972713\t8.893700\t-0.420783\t0.494041\t-123.316913\t0.507000\t0.002000\n\t\n15:50:59.4\tlog_raw\tgps_raw\t#DUALANTENNAHEADINGA,USB3,0,43.5,FINESTEERING,2107,283877.400,02000000,d426,15824;INSUFFICIENT_OBS,NONE,-1.000000000,0.000000000,0.000000000,0.0,0.000000000,0.000000000,\"631T\",12,3,3,3,04,00,20,00*231fd75a\n\tsystem status\tnormal 2 27.800000 0 0\trobot status\t45.895976\t60.784930\t8.897900\t-0.492737\t0.506162\t-123.287108\t0.552000\t-0.092000\n\t\n15:50:59.9\tlog_raw\tgps_raw\t#INSPVAXA,USB3,0,43.5,FINESTEERING,2107,283877.900,02000000,471d,15824;INS_ALIGNMENT_COMPLETE,INS_RTKFIXED,37.37067617157,126.72135158509,8.9007,22.3000,-0.3585,-0.2879,0.0250,-0.387485023,0.488203983,213.381189141,0.4358,0.3051,0.6016,0.1150,0.0957,0.0873,0.0971,0.1009,5.1472,0f000001,0*c9483ecc\n\tsystem status\tnormal 2 27.800000 0 0\trobot status\t45.748952\t60.594697\t8.900700\t-0.387485\t0.488204\t-123.381189\t0.483000\t0.005000\n\t\n15:51:00.4\tlog_raw\tgps_raw\t#DUALANTENNAHEADINGA,USB3,0,49.5,FINESTEERING,2107,283878.400,02000000,d426,15824;INSUFFICIENT_OBS,NONE,-1.000000000,0.000000000,0.000000000,0.0,0.000000000,0.000000000,\"631T\",9,3,3,3,04,00,20,00*27e46637\n\tsystem status\tnormal 2 27.800000 0 0\trobot status\t45.606127\t60.408915\t8.905900\t-0.330254\t0.526641\t-123.363969\t0.502000\t0.007000\n\t\n15:51:00.9\tlog_raw\tgps_raw\t#INSPVAXA,USB3,0,49.5,FINESTEERING,2107,283878.900,02000000,471d,15824;INS_ALIGNMENT_COMPLETE,INS_RTKFIXED,37.37067289269,126.72134842166,8.9107,22.3000,-0.2321,-0.2053,0.0305,-0.361897679,0.347183543,213.363814143,0.4356,0.3048,0.6022,0.1141,0.0948,0.0861,0.0972,0.1010,5.1487,0f000001,0*7c1228c2\n\tsystem status\tnormal 2 27.800000 0 0\trobot status\t45.468741\t60.230793\t8.910700\t-0.361898\t0.347184\t-123.363814\t0.262000\t0.102000\n\t\n15:51:01.4\tlog_raw\tgps_raw\t#INSPVAXA,USB3,0,50.0,FINESTEERING,2107,283879.400,02000000,471d,15824;INS_ALIGNMENT_COMPLETE,INS_RTKFIXED,37.37067136914,126.72134696073,8.9138,22.3000,-0.4356,-0.3421,0.0457,-0.368595541,0.477690460,213.236251513,0.4352,0.3048,0.6024,0.1137,0.0954,0.0849,0.0973,0.1011,5.1500,0f000001,0*de91db37\n\tsystem status\tnormal 2 27.700000 0 0\trobot status\t45.339334\t60.061703\t8.913800\t-0.368596\t0.477690\t-123.236252\t0.536000\t-0.002000\n\t\n15:51:01.9\tlog_raw\tgps_raw\t#DUALANTENNAHEADINGA,USB3,0,50.0,FINESTEERING,2107,283879.900,02000000,d426,15824;INSUFFICIENT_OBS,NONE,-1.000000000,0.000000000,0.000000000,
